vi "not forget.vi"() -> ()   [LabVIEW 2018]
uses:
  <instrlib>/Rohde&Schwarz RF Signal Generator/Rohde&Schwarz RF Signal Generator.lvlib
panel:
  in  "MW_Parameters":T1
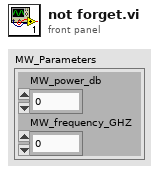
[diagram p1: front panel]
types:
  T1 = cluster{"MW_power_db":dbl, "MW_frequency_GHZ":dbl}
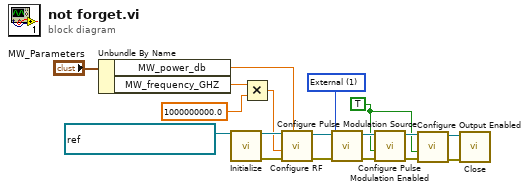
[diagram p0: block diagram]
diagram:
  w8 = 1 items=["Internal", "External", "Coder"] ("Source (Internal)")
  w1 = TRUE ("Pulse Modulation Enabled (Off)")
  n1 = Unbundle By Name("MW_Parameters") -> ("MW_power_db"=w12:dbl, "MW_frequency_GHZ"=w11:dbl)
  n2 = call <instrlib>:"Initialize.vi"("VISA resource name"=refnum<visa-resource-name> refnum) -> ("VISA resource name out"=w16:refnum<visa-resource-name>, "error out"=w15:errorcluster)  [unwired: 13 in]
  n3 = Multiply(x=w11, y=1000000000.0) -> (x*y=w9:dbl)
  n4 = call <instrlib>:"Configure RF.vi"("Power Level (-30.0)"=w12, "error in (no error)"=w15, "Frequency (1GHz)"=w9, "VISA resource name"=w16) -> ("error out"=w17:errorcluster, "VISA resource name out"=w18:refnum<visa-resource-name>)  [unwired: 6 in]
  n5 = call <instrlib>:"Configure Pulse Modulation Source.vi"("error in (no error)"=w17, "Source (Internal)"=w8, "VISA resource name"=w18) -> ("error out"=w7:errorcluster, "VISA resource name out"=w6:refnum<visa-resource-name>)  [unwired: 7 in]
  n6 = call <instrlib>:"Configure Pulse Modulation Enabled.vi"("error in (no error)"=w7, "Pulse Modulation Enabled (Off)"=w1, "VISA resource name"=w6) -> ("error out"=w4:errorcluster, "VISA resource name out"=w5:refnum<visa-resource-name>)  [unwired: 7 in]
  n7 = call <instrlib>:"Configure Output Enabled.vi"("error in (no error)"=w4, "Output Enabled (Off)"=w1, "VISA resource name"=w5) -> ("error out"=w2:errorcluster, "VISA resource name out"=w3:refnum<visa-resource-name>)  [unwired: 7 in]
  n8 = call <instrlib>:"Close.vi"("error in (no error)"=w2, "VISA resource name"=w3) -> ()  [unwired: 9 in, 1 out]
